vi "niFPGA BFGroup Twiddle Table 8 U32.vi"(7 "address":fxp<+,3,3>) -> (4 "twid real":fxp<+/-,17,2> format="%.16g", 6 "twid imag":fxp<+/-,17,2> format="%.16g")   [LabVIEW 2017]
uses:
  <vilib>/rvi/FXPMathLib/basic elements/FxpDiscreteDelay/XNode/nifxpmath_DiscreteDelay.xnode
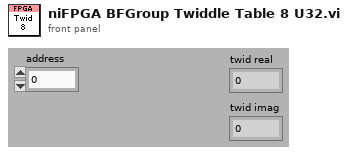
[diagram p1: front panel]
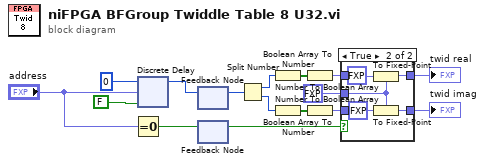
[diagram p0: block diagram]
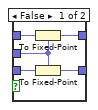
[diagram p2: hidden frame]
diagram:
  n1 = Equal To 0?(x="address") -> (x = 0?=w7:bool)
  n2 = xnode "Discrete Delay"("D"=u32 0, "n-1[0..15]"="address", "enable"=FALSE) -> ("Q"=w1:u32)
  n3 = feedback-in #1(w1) -> ()
  n4 = feedback #1() -> (w12:u32)  [unwired: 1 out]
  n5 = feedback-in #2(w7) -> ()
  n6 = feedback #2() -> (w6:bool)  [unwired: 1 out]
  n7 = Split Number(x=w12) -> (hi(x)=w15:u16, lo(x)=w13:u16)
  n8 = Number To Boolean Array(number=w15) -> (Boolean array=w16:bool[])
  n9 = Number To Boolean Array(number=w13) -> (Boolean array=w14:bool[])
  n10 = Boolean Array To Number(Boolean array=w16) -> (number=w11:fxp<+/-,16,1>)
  n11 = Boolean Array To Number(Boolean array=w14) -> (number=w9:fxp<+/-,16,1>)
  n12 = case shown="True" w6 {
    tunnel: w11 -> [w21 _]
    tunnel: [w20 w26] -> w10
    tunnel: w9 -> [w19 _]
    tunnel: [w18 w23] -> w8
    tunnel: fxp<+/-,17,2> 0.0 ("fixed-point type") -> [w17 w22]
    frame False {
      n13 = To Fixed-Point(fixed-point type=w17, number=w21) -> (fixed-point=w20:fxp<+/-,17,2>)
      n14 = To Fixed-Point(fixed-point type=w17, number=w19) -> (fixed-point=w18:fxp<+/-,17,2>)
    }
    frame True {
      n15 = To Fixed-Point(fixed-point type=w22, number=fxp<+,1,1> 1.0 ("fixed-point type")) -> (fixed-point=w26:fxp<+/-,17,2>)
      n16 = To Fixed-Point(fixed-point type=w22, number=fxp<+,1,1> 0.0 ("fixed-point type")) -> (fixed-point=w23:fxp<+/-,17,2>)
    }
  }
  "twid real" <- w10
  "twid imag" <- w8
